vi "Fichero_create.vi"(8 "error in (no error)":errorcluster, 9 "formato":string, 10 "Nombre Fichero":string, 11 "Direccion":path) -> (0 "error out":errorcluster, 3 "Byte Stream File out":refnum<file>)   [LabVIEW 2020]
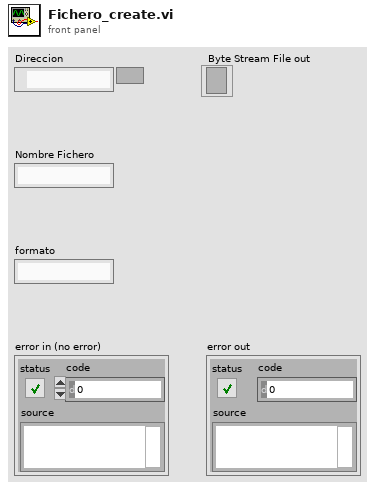
[diagram p1: front panel]
types:
  T1 = enum16{"open", "replace", "create", "open or create", "replace or create", "replace or create with confirmation"}
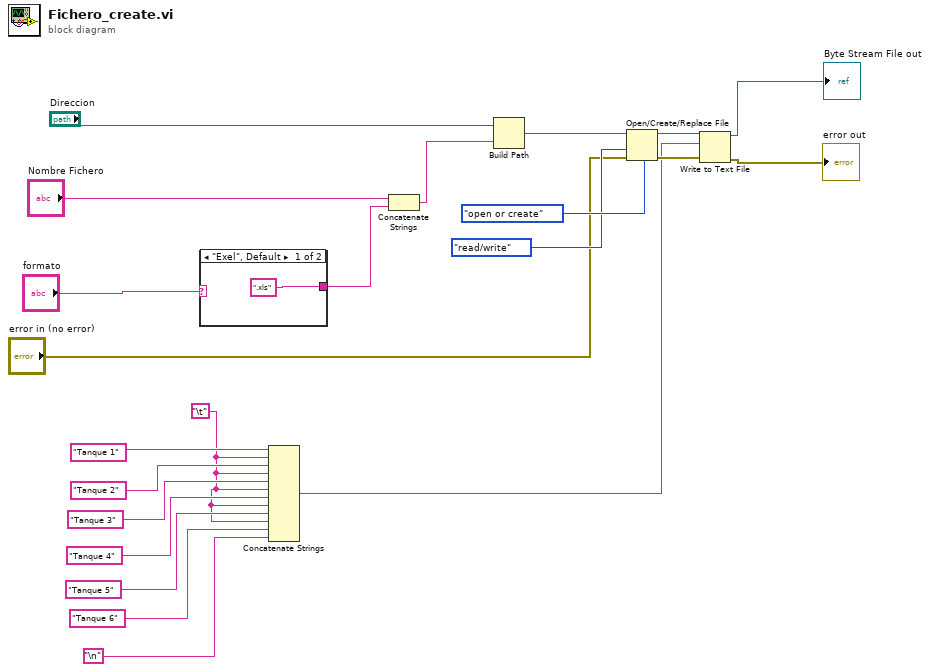
[diagram p0: block diagram]
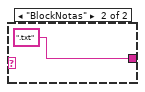
[diagram p2: hidden frame]
diagram:
  w2 = "\t"
  n1 = case shown="\"Exel\", Default" "formato" {
    tunnel: [".xls" ".txt"] -> w12
    frame "Exel", Default {
    }
    frame "BlockNotas" {
    }
  }
  n2 = Concatenate Strings("Tanque 1", w2, "Tanque 2", w2, "Tanque 3", w2, "Tanque 4", w2, "Tanque 5", w2, "Tanque 6", "\n") -> (w9:string)
  n3 = Concatenate Strings("Nombre Fichero", w12) -> (w13:string)
  n4 = Build Path(base path="Direccion", name or relative path=w13) -> (appended path=w15:path)
  n5 = Open/Create/Replace File(file path (use dialog)=w15, error in="error in (no error)", operation (0:open)=T1."open or create", access (0:read/write)=enum16{"read/write", "read-only", "write-only"}."read/write") -> (refnum out=w19:refnum<file>, error out=w20:errorcluster)  [unwired: 2 in, 1 out]
  n6 = Write to Text File(file (use dialog)=w19, text=w9, error in=w20) -> (refnum out=→"Byte Stream File out":refnum<file>, error out=→"error out":errorcluster)  [unwired: 1 in, 1 out]
